vi "display permission to classification.vi"(11 "display permissions":T1) -> (3 "channel classification":T2)   [LabVIEW 2013, in "Modbus Slave editor node.lvclass"]
doc: "Platypus Framework 1.0.1.65\nNI Systems Engineering - National Instruments"
uses:
  Modbus Slave editor node.lvclass
  <vilib>/NI/Tag Bus Module Framework/channel/channel classification.ctl
  <vilib>/NI/Tag Bus Module Framework/channel/TBM channel.lvclass
  permissions.ctl
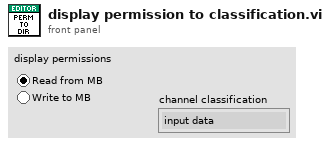
[diagram p1: front panel]
types:
  T1 = typedef "Modbus Slave editor node.lvclass/permissions.ctl" = enum32{"Read from MB", "Write to MB"}
  T2 = typedef "TBM channel.lvclass/channel classification.ctl" = enum16{"input data", "output data", "processing parameter", "processing result"}
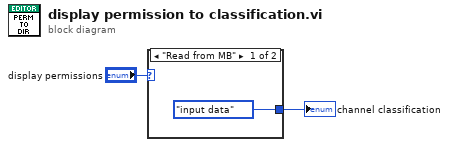
[diagram p0: block diagram]
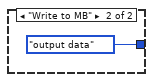
[diagram p2: hidden frame]
diagram:
  n1 = case shown="\"Read from MB\"" "display permissions" {
    tunnel: [channel_classification."input data" ("channel classification") channel_classification."output data" ("channel classification")] -> w2
    frame "Read from MB" {
    }
    frame "Write to MB" {
    }
  }
  "channel classification" <- w2
